vi "Init Client.vi"(7 "Client TLS Config (Disabled)":T1, 8 "error in (no error)":errorcluster, 9 "local-port":u16 caption="local-port (0=any)", 10 "Port":u16, 11 "Host":string) -> (0 "error out":errorcluster, 3 "TinyTCP Client":T3)   [LabVIEW 2020, in "TinyTCP.lvlib"]
doc: "Initializes a TCP Client that will connect to the specified server once <b>Open.vi</b> is called. Once Open is called, the client will continually attempt to connect to the server and if connection is lost it will reconnect. The status of the connection can be checked with <b>Get State.vi</b> Once the connection is no longer needed, call <b>Close.vi</b> to close the client connection. To cleanup the client and release all resources call <b>Stop.vi</b>\n\nA Client TLS Config can optionally be specified to enable and enforce TLS handshakes when connecting. This will cause all data to be encrypted sent via the connection. If the Server being connected to uses a different name in its certificate then the Host value used to establish the client connection, be sure to include the expected Server Name that will be listed in the server certificate that the TLS handshake validates.\n\nFor local port, if the value is 0, the operating system selects an unused port. The default is 0."
uses:
  TinyTCP.lvlib
  Instance.ctl
  Ref Data.ctl
  State.ctl
  Client TLS Config.ctl
  Cert Chain.ctl
  TLS Config.ctl
panel:
  # "If the value is 0, the operating system selects an unused port. The default is 0."
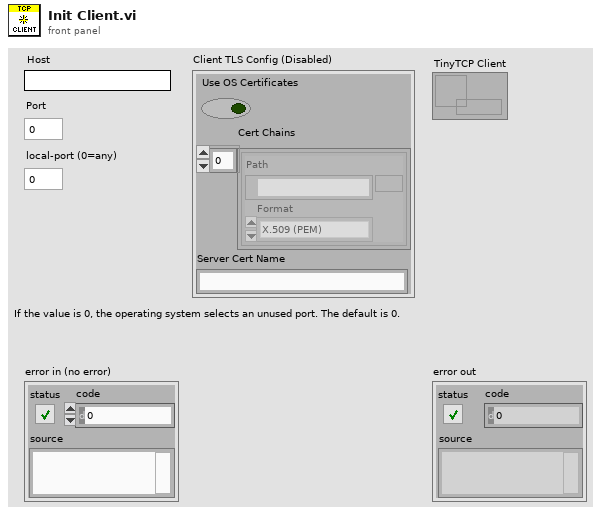
[diagram p1: front panel]
types:
  T1 = typedef "TinyTCP.lvlib/Client TLS Config.ctl" = cluster{"Use OS Certificates":bool, "Cert Chains":T2[], "Server Cert Name":string}
  T2 = typedef "TinyTCP.lvlib/Cert Chain.ctl" = cluster{"Path":path, "Format":enum32{"X.509 (PEM)"}}
  T3 = typedef "TinyTCP.lvlib/Instance.ctl" = refnum<data-value>
  T4 = typedef "TinyTCP.lvlib/TLS Config.ctl" = cluster{"TLS Enabled":bool, "Use OS Cert Chains":bool, "Private Key Path":path, "Private Key Format":enum32{"PKCS#8 (PEM)", "PKCS#8 (DER)"}, "Private Key Password":string, "Private Key Cert Chain":T2, "Cert Chains":T2[]}
  T5 = typedef "TinyTCP.lvlib/Ref Data.ctl" = cluster{"TCP":refnum<k5>, "State":T6, "Server":bool, "Host":string, "Port":u16, "Listener":refnum<k5>, "Start":bool, "Disconnect":bool, "TCP Valid":bool, "TLS Enabled":bool, "Immutable TLS":refnum<k36>, "Certificate DN":string, "local-port":u16}
  T6 = typedef "TinyTCP.lvlib/State.ctl" = enum16{"Idle", "Starting", "Connecting", "Connected", "Disconnecting", "Stopped"}
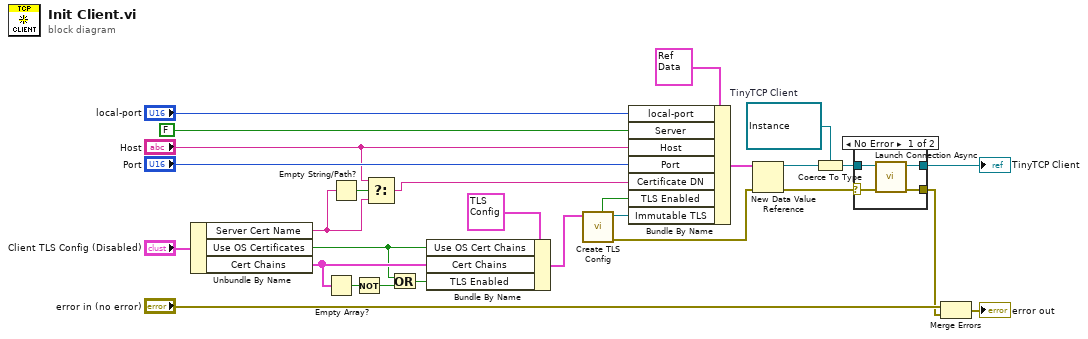
[diagram p0: block diagram]
diagram:
  w22 = T3 refnum  # TinyTCP Client
  n1 = Unbundle By Name("Client TLS Config (Disabled)") -> ("Server Cert Name"=w8:string, "Use OS Certificates"=w10:bool, "Cert Chains"=w14:T2[])
  n2 = Empty Array?(array=w14) -> (empty?=w13:bool)
  n3 = Empty String/Path?(string/path=w8) -> (empty?=w9:bool)
  n4 = Not(x=w13) -> (.not. x?=w12:bool)
  n5 = Select(t="Host", s=w9, f=w8) -> (s? t:f=w6:string)
  n6 = Or(x=w10, y=w12) -> (x .or. y?=w11:bool)
  n7 = Bundle By Name(cluster=T4 {"TLS Enabled"=FALSE, "Use OS Cert Chains"=FALSE, "Private Key Path"=path "", "Private Key Format"=enum."PKCS#8 (PEM)", "Private Key Password"="", "Private Key Cert Chain"={"Path"=path "", "Format"=enum."X.509 (PEM)"}, "Cert Chains"=[]} ("TLS Config"), "Use OS Cert Chains"=w10, "Cert Chains"=w14, "TLS Enabled"=w11) -> (w15:T4)
  n8 = call "Create TLS Config.vi"("TLS Config"=w15) -> ("error out"=w18:errorcluster, "Immutable TLS"=w20:refnum<k36>, "TLS Enabled"=w19:bool)  [unwired: 8 in]
  n9 = Bundle By Name(cluster=T5 {"TCP"=refnum, "State"=enum."Idle", "Server"=FALSE, "Host"="", "Port"=0, "Listener"=refnum, "Start"=FALSE, "Disconnect"=FALSE, "TCP Valid"=FALSE, "TLS Enabled"=FALSE, "Immutable TLS"=refnum, "Certificate DN"="", "local-port"=0} ("Ref Data"), "local-port"="local-port", "Server"=FALSE, "Host"="Host", "Port"="Port", "Certificate DN"=w6, "TLS Enabled"=w19, "Immutable TLS"=w20) -> (w26:T5)
  n10 = New Data Value Reference(data value=w26, error in=w18) -> (data value reference=w23:refnum<data-value>, error out=w3:errorcluster)
  n11 = Coerce To Type(0:w23, 1:w22) -> (2:w5:T3)
  n12 = case shown="No Error" w3 {
    selector: w3 -> [w30 w33]
    tunnel: w5 -> [w32 w34]
    tunnel: [w31 w34] -> w4
    tunnel: [w29 w33] -> w2
    frame No Error {
      n13 = call "Launch Connection Async.vi"("error in (no error)"=w30, "TCP Comm In"=w32) -> ("error out"=w29:errorcluster, "TCP Comm"=w31:T3)  [unwired: 8 in]
    }
    frame Error {
    }
  }
  "TinyTCP Client" <- w4
  n14 = Merge Errors("error in (no error)", w2) -> (→"error out":errorcluster)
